vi "TL4000 Set Output Protection Voltage.vi"(8 "error in (no error)":errorcluster {"code" format="%.0x"}, 10 "Voltage (5.0)":dbl=5.0, 11 "instrument handle":refnum<visa-resource-name>) -> (0 "error out":errorcluster {"code" format="%.0x"}, 3 "instrument handle out":refnum<visa-resource-name>)   [LabVIEW 2019]
doc: "This VI sets the laser output protection voltage.\n\nNote: \nThis VI is valid for: LDC4000, ITC4000"
uses:
  TL4000_32.dll
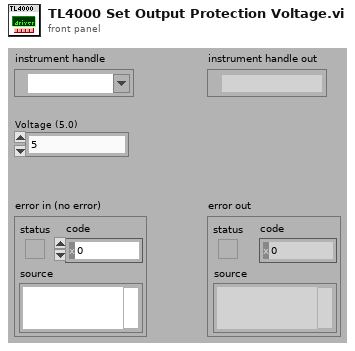
[diagram p1: front panel]
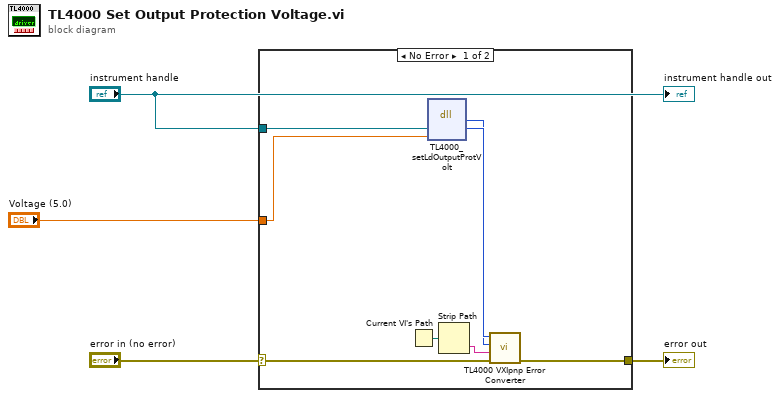
[diagram p0: block diagram]
diagram:
  n1 = case shown="No Error" "error in (no error)" {
    selector: "error in (no error)" -> [w7 w13]
    tunnel: [w6 w13] -> w4
    tunnel: "instrument handle" -> [w11 _]
    tunnel: "Voltage (5.0)" -> [w5 _]
    frame No Error {
      n2 = Current VI's Path() -> (path=w12:path)
      n3 = dll-call lib="TL4000_32.*" fn="TL4000_setLdOutputProtVolt"("Instrument Handle"=w11, "Voltage"=w5) -> (w9:i32, "Instrument Handle"=w10:u32)  [unwired: 4 in, 2 out]
      n4 = Strip Path(path=w12) -> (name=w8:string)  [unwired: 1 out]
      n5 = call "TL4000 VXIpnp Error Converter.vi"("error in (no error)"=w7, "Name Of VI (\"\")"=w8, "CVI Error Code (0)"=w9, "instrument handle"=w10) -> ("error out"=w6:errorcluster)  [unwired: 6 in, 1 out]
    }
    frame Error {
    }
  }
  "error out" <- w4
  "instrument handle out" <- "instrument handle"
